vi "GOMDBTS2048 calib Tristimulus Get XYZ.vi"(8 "error in (no error)":errorcluster, 11 "handle":i32) -> (0 "error out":errorcluster, 1 "valuesZ":dbl[](array[numeric]), 2 "valuesY":dbl[](array[numeric]), 3 "valuesX":dbl[](array[numeric]), 5 "function return":i32)   [LabVIEW 2015, in "GOMDBTS2048.lvlib"]
doc: "GOBTS2048DLL int __stdcall GOMDBTS2048_calibTristimulusSetXYZ(int handle, double* valuesX, double* valuesY, double* valuesZ); GOBTS2048DLL int __stdcall GOMDBTS2048_calibTristimulusGetXYZ(int handle, double* valuesX, double* valuesY, double* valuesZ);"
uses:
  GOMDBTS2048.lvlib
  runtime/GOMDBTS2048.dll
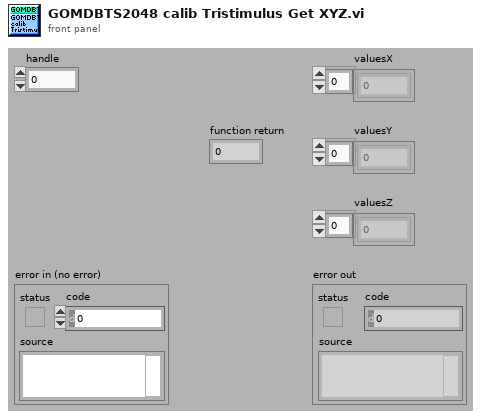
[diagram p1: front panel]
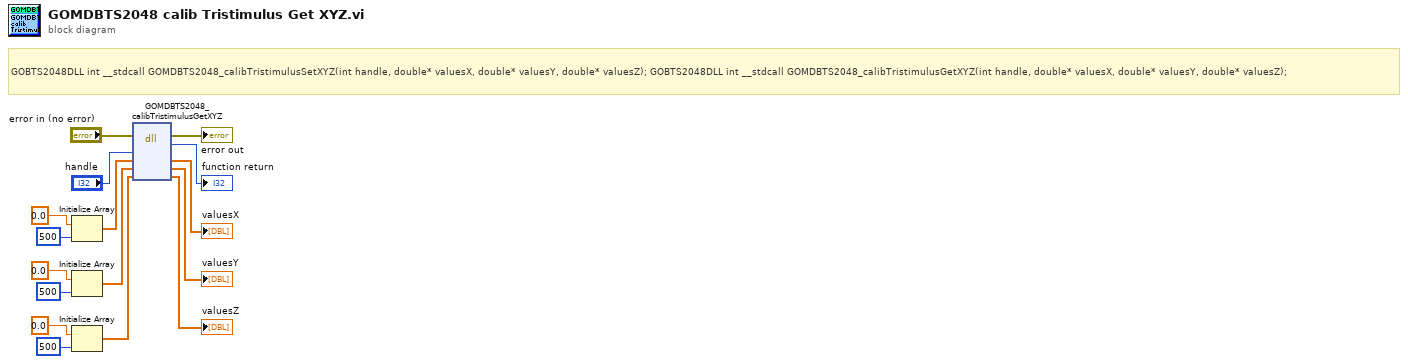
[diagram p0: block diagram]
diagram:
  # "GOBTS2048DLL int __stdcall GOMDBTS2048_calibTristimulusSetXYZ(int handle, double* valuesX, double* valuesY, double* valuesZ); GOBTS2048DLL int __stdcall GOMDBTS2048_calibTristimulusGetXYZ(int handle, double* valuesX, double* valuesY, double* valuesZ);"
  n1 = Initialize Array(0.0 ("element"), 500 ("dimension size")) -> (w14:dbl[])
  n2 = Initialize Array(0.0 ("element"), 500 ("dimension size")) -> (w10:dbl[])
  n3 = Initialize Array(0.0 ("element"), 500 ("dimension size")) -> (w6:dbl[])
  n4 = dll-call lib="C:/Users/rkoch/Documents/GO_Library/runtime/GOMDBTS2048.*" fn="GOMDBTS2048_calibTristimulusGetXYZ"(error in="error in (no error)", "handle"="handle", "valuesX"=w14, "valuesY"=w10, "valuesZ"=w6) -> (error out=→"error out":errorcluster, →"function return":i32, "valuesX"=→"valuesX":dbl[], "valuesY"=→"valuesY":dbl[], "valuesZ"=→"valuesZ":dbl[])  [unwired: 3 in, 1 out]
